vi "DiscoveryProtoTest.vi"() -> ()   [LabVIEW 2020, in "VectoScratch.lvlib"]
uses:
  VectoScratch.lvlib
  Vecto/proto/Discovery/Data.ctl
  Vecto/proto/Service/Data.ctl
  Vecto/proto/ServiceType/Enumeration.ctl
  Vecto/proto/Discovery/Discovery.lvlib
  Vecto/proto/ServiceType/ServiceType.lvlib
  Vecto/proto/Service/Service.lvlib
panel:
  out "Data":T1={"node_id"=0, "name"="Gamma", "ip"=170583000, "status"="Undefined", "services"=[{"type"=enum."SERVICETYPE_HTTPSERVER", "port"=36985}], "system"="", "cluster"="", "app_version"="", "cfg_version"=""}
  out "error out":errorcluster
  out "string":string
  in  "Discovery":T1={"node_id"=0, "name"="Gamma", "ip"=170583000, "status"="Undefined", "services"=[{"type"=enum."SERVICETYPE_HTTPSERVER", "port"=36985}], "system"="", "cluster"="", "app_version"="", "cfg_version"=""}
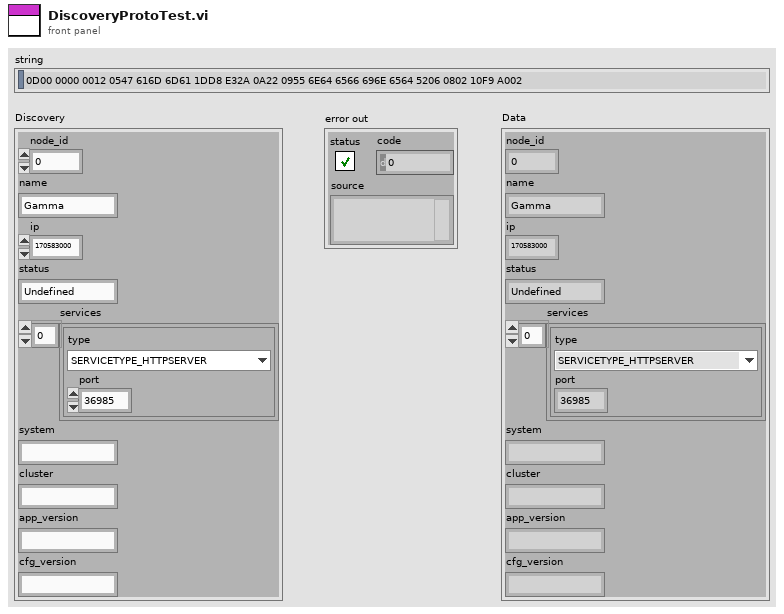
[diagram p1: front panel]
types:
  T1 = typedef "Discovery.lvlib/Data.ctl" = cluster{"node_id":u32, "name":string, "ip":u32, "status":string, "services":T2[], "system":string, "cluster":string, "app_version":string, "cfg_version":string}
  T2 = typedef "Service.lvlib/Data.ctl" = cluster{"type":T3, "port":i32}
  T3 = typedef "ServiceType.lvlib/Enumeration.ctl" = enum16{"SERVICETYPE_UNKNOWN", "SERVICETYPE_TCPSERVER", "SERVICETYPE_HTTPSERVER"}
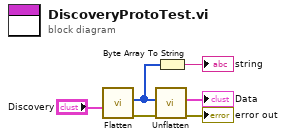
[diagram p0: block diagram]
diagram:
  n1 = call "Flatten.vi"("Data"="Discovery") -> ("error out"=w3:errorcluster, "Buffer"=w4:u8[])  [unwired: 9 in]
  n2 = call "Unflatten.vi"("error in"=w3, "Buffer"=w4) -> ("error out"=→"error out":errorcluster, "Data"=→"Data":T1)  [unwired: 8 in]
  n3 = Byte Array To String(unsigned byte array=w4) -> (string=→"string":string)
